vi "StreamReceiveTCS.vi"() -> ()   [LabVIEW 2018]
panel:
  out "error out":errorcluster
  in  "stop 2":bool
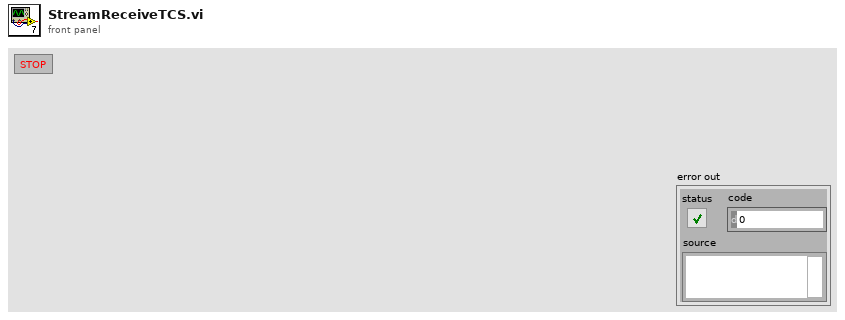
[diagram p1: front panel]
types:
  T1 = enum16{"Standard", "Buffered", "CRLF", "Immediate"}
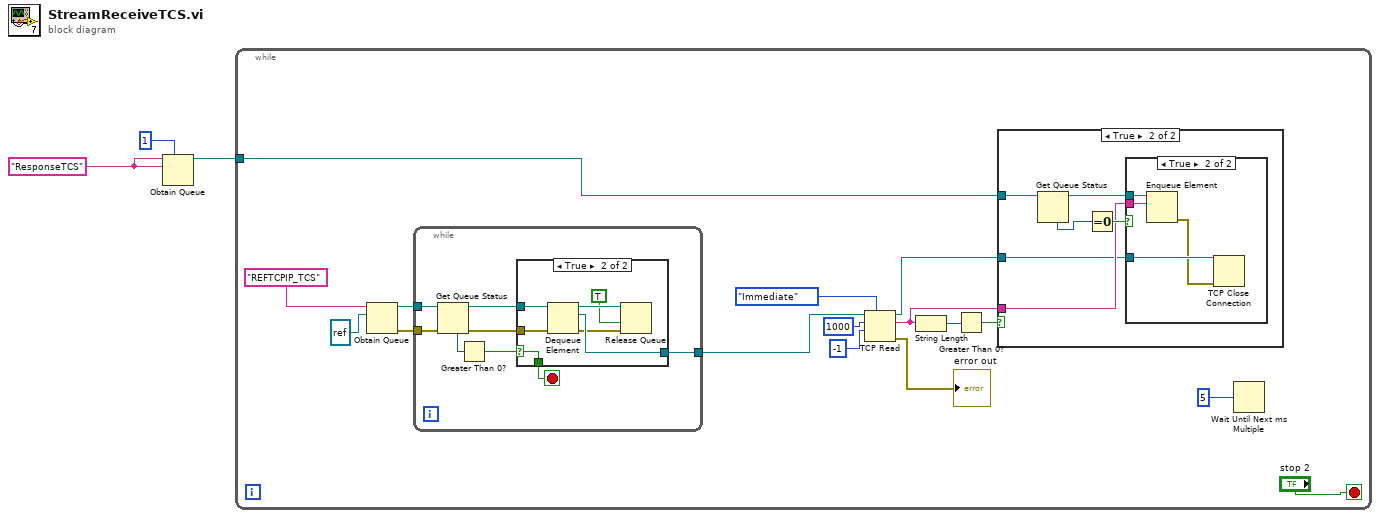
[diagram p0: block diagram]
diagram:
  w3 = "ResponseTCS"
  n1 = Obtain Queue(max queue size (-1, unlimited)=1, name (unnamed)=w3, element data type=w3) -> (queue out=w2:refnum<queue>)  [unwired: 2 in, 2 out]
  n2 = while {
    tunnel: w2 -> [w19]
    stop <- "stop 2" stop-if-true
    n3 = Obtain Queue(name (unnamed)="REFTCPIP_TCS", element data type=refnum<k5> refnum ("connection ID out 2")) -> (queue out=w16:refnum<queue>, error out=w15:errorcluster)  [unwired: 3 in, 1 out]
    n4 = while {
      tunnel: [w37] -> w18
      tunnel: w16 -> [w36]
      tunnel: w15 -> [w33]
      stop <- w30 stop-if-true
      n5 = Get Queue Status(queue=w36, error in (no error)=w33) -> (queue out=w35:refnum<queue>, error out=w34:errorcluster, # elements in queue=w31:i32)  [unwired: 1 in, 5 out]
      n6 = Greater Than 0?(x=w31) -> (x > 0?=w32:bool)
      n7 = case shown="True" w32 {
        selector: w32 -> [w38 w42]
        tunnel: [_ w45] -> w37
        tunnel: w35 -> [_ w44]
        tunnel: w34 -> [_ w43]
        tunnel: [w38 w42] -> w30
        frame False {
        }
        frame True {
          n8 = Dequeue Element(queue=w44, error in (no error)=w43) -> (queue out=w41:refnum<queue>, element=w45:refnum<k5>, error out=w40:errorcluster)  [unwired: 1 in, 1 out]
          n9 = Release Queue(queue=w41, force destroy? (F)=TRUE, error in (no error)=w40) -> ()  [unwired: 3 out]
        }
      }
    }
    n10 = TCP Read(connection ID=w18, bytes to read=1000, 7:T1."Immediate" ("mode (standard)"), 9:-1 ("bytes to read")) -> (connection ID out=w6:refnum<k5>, data out=w11:string, error out=→"error out":errorcluster)  [unwired: 1 in]
    n11 = String Length(string=w11) -> (length=w13:i32)
    n12 = Greater Than 0?(x=w13) -> (x > 0?=w12:bool)
    n13 = case shown="True" w12 {
      tunnel: w19 -> [_ w23]
      tunnel: w11 -> [_ w21]
      tunnel: w6 -> [_ w20]
      frame False {
      }
      frame True {
        n14 = Get Queue Status(queue=w23) -> (queue out=w22:refnum<queue>, # elements in queue=w25:i32)  [unwired: 2 in, 6 out]
        n15 = Equal To 0?(x=w25) -> (x = 0?=w24:bool)
        n16 = case shown="True" w24 {
          tunnel: w22 -> [_ w29]
          tunnel: w21 -> [_ w28]
          tunnel: w20 -> [_ w27]
          frame False {
          }
          frame True {
            n17 = Enqueue Element(queue=w29, element=w28) -> (error out=w26:errorcluster)  [unwired: 2 in, 2 out]
            n18 = TCP Close Connection(connection ID=w27, error in (no error)=w26) -> ()  [unwired: 1 in, 2 out]
          }
        }
      }
    }
    n19 = Wait Until Next ms Multiple(millisecond multiple=u32 5) -> ()  [unwired: 1 out]
  }
